vi "Write Session.TCPIP.KeepAliveInterval.vi"(8 "error in (no error)":errorcluster, 10 "Session.TCPIP.KeepAliveInterval":dbl, 11 "SLSC Remote in":refnum<class "SLSC Remote.lvclass">) -> (0 "error out":errorcluster, 3 "SLSC Remote out":refnum<class "SLSC Remote.lvclass">)   [LabVIEW 2015, in "SLSC Remote.lvclass"]
uses:
  SLSC Remote.lvclass
  SLSC Interface Class/SLSC Interface.lvclass
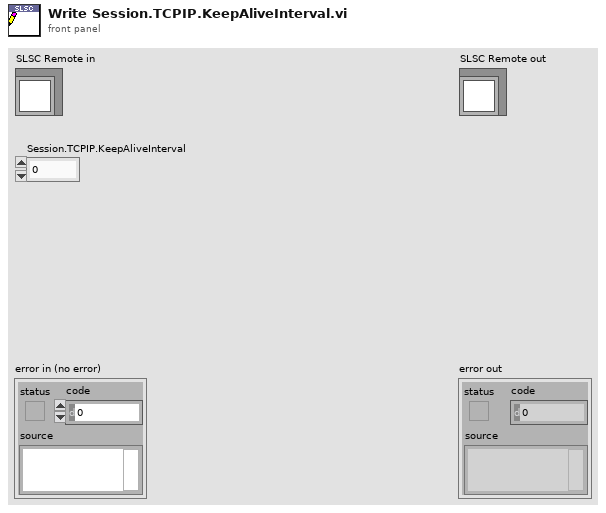
[diagram p1: front panel]
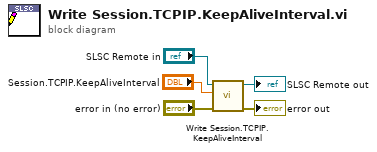
[diagram p0: block diagram]
diagram:
  n1 = call-parent "Write Session.TCPIP.KeepAliveInterval.vi"("error in (no error)"="error in (no error)", "Session.TCPIP.KeepAliveInterval"="Session.TCPIP.KeepAliveInterval", "SLSC Interface in"="SLSC Remote in") -> ("error out"=→"error out":errorcluster, "SLSC Interface out"=→"SLSC Remote out":refnum<class "SLSC Remote.lvclass">)  [unwired: 7 in]
